vi "day 16 task 1.vi"   [LabVIEW 2019]
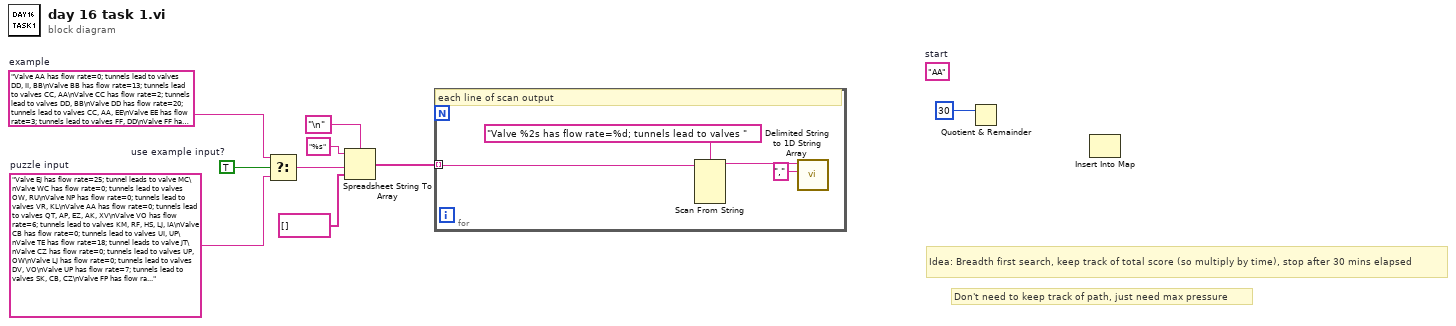
[diagram p0: block diagram]
diagram:
  (unwired) "AA"  # start
  w3 = TRUE  # use example input?
  w4 = "Valve EJ has flow rate=25; tunnel leads to valve MC\nValve WC has flow rate=0; tunnels lead to valves OW, RU\nValve NP has flow rate=0; tunnels lead to valves VR, KL\nValve AA has flow rate=0; tunnels lead to valves QT, AP, EZ, AK, XV\nValve VO has flow rate=6; tunnels lead to valves KM, RF, HS, LJ, IA\nValve CB has flow rate=0; tunnels lead to valves UI, UP\nValve TE has flow rate=18; tunnel leads to valve JT\nValve CZ has flow rate=0; tunnels lead to valves UP, OW\nValve LJ has flow rate=0; tunnels lead to valves DV, VO\nValve UP has flow rate=7; tunnels lead to valves SK, CB, CZ\nValve FP has flow rate=0; tunnels lead to valves OW, RE\nValve KM has flow rate=0; tunnels lead to valves SE, VO\nValve DV has flow rate=0; tunnels lead to valves LJ, UM\nValve FL has flow rate=0; tunnels lead to valves AH, TS\nValve VR has flow rate=24; tunnels lead to valves DM, TF, NP\nValve IA has flow rate=0; tunnels lead to valves VS, VO\nValve RF has flow rate=0; tunnels lead to valves VO, JF\nValve RT has flow rate=0; tunnels lead to valves UM, SE\nValve RU has flow rate=0; tunnels lead to valves AR, WC\nValve SE has flow rate=4; tunnels lead to valves GU, KM, CX, RT\nValve MC has flow rate=0; tunnels lead to valves EJ, AR\nValve TF has flow rate=0; tunnels lead to valves AH, VR\nValve CX has flow rate=0; tunnels lead to valves SE, TO\nValve GL has flow rate=11; tunnels lead to valves UY, KL, CY\nValve GU has flow rate=0; tunnels lead to valves SE, EZ\nValve VS has flow rate=0; tunnels lead to valves XN, IA\nValve EZ has flow rate=0; tunnels lead to valves AA, GU\nValve GK has flow rate=0; tunnels lead to valves FI, HZ\nValve JT has flow rate=0; tunnels lead to valves TE, XN\nValve DM has flow rate=0; tunnels lead to valves VR, HZ\nValve AR has flow rate=16; tunnels lead to valves UI, RU, MC\nValve XN has flow rate=9; tunnels lead to valves XP, JT, VS, GT, CY\nValve CY has flow rate=0; tunnels lead to valves XN, GL\nValve QT has flow rate=0; tunnels lead to valves UM, AA\nValve KL has flow rate=0; tunnels lead to valves GL, NP\nValve SK has flow rate=0; tunnels lead to valves XV, UP\nValve OW has flow rate=12; tunnels lead to valves CZ, WC, FP\nValve AK has flow rate=0; tunnels lead to valves AA, HS\nValve XV has flow rate=0; tunnels lead to valves AA, SK\nValve GT has flow rate=0; tunnels lead to valves XN, UM\nValve FI has flow rate=0; tunnels lead to valves JF, GK\nValve UY has flow rate=0; tunnels lead to valves JF, GL\nValve UM has flow rate=5; tunnels lead to valves DV, GT, RT, QT\nValve IQ has flow rate=0; tunnels lead to valves HZ, AH\nValve JF has flow rate=10; tunnels lead to valves RF, FI, UY, RE, TS\nValve TS has flow rate=0; tunnels lead to valves JF, FL\nValve AH has flow rate=23; tunnels lead to valves IQ, FL, TF\nValve HS has flow rate=0; tunnels lead to valves AK, VO\nValve HZ has flow rate=20; tunnels lead to valves IQ, DM, GK\nValve TO has flow rate=15; tunnel leads to valve CX\nValve XP has flow rate=0; tunnels lead to valves AP, XN\nValve AP has flow rate=0; tunnels lead to valves XP, AA\nValve RE has flow rate=0; tunnels lead to valves JF, FP\nValve UI has flow rate=0; tunnels lead to valves AR, CB"  # puzzle input
  w5 = "Valve AA has flow rate=0; tunnels lead to valves DD, II, BB\nValve BB has flow rate=13; tunnels lead to valves CC, AA\nValve CC has flow rate=2; tunnels lead to valves DD, BB\nValve DD has flow rate=20; tunnels lead to valves CC, AA, EE\nValve EE has flow rate=3; tunnels lead to valves FF, DD\nValve FF has flow rate=0; tunnels lead to valves EE, GG\nValve GG has flow rate=0; tunnels lead to valves FF, HH\nValve HH has flow rate=22; tunnel leads to valve GG\nValve II has flow rate=0; tunnels lead to valves AA, JJ\nValve JJ has flow rate=21; tunnel leads to valve II"  # example
  # "Don't need to keep track of path, just need max pressure"
  # "Idea: Breadth first search, keep track of total score (so multiply by time), stop after 30 mins elapsed"
  n1 = Select(t=w5, s=w3, f=w4) -> (s? t:f=w2:string)
  n2 = Spreadsheet String To Array(delimiter (Tab)="\n", format string="%s", spreadsheet string=w2, array type (2D Dbl)=string[] []) -> (array=w6:string[])
  n3 = for {
    tunnel: w6 -> [w13] mode=indexing
    # "each line of scan output"
    n4 = Scan From String(format string="Valve %2s has flow rate=%d; tunnels lead to valves ", input string=w13) -> (remaining string=w11:string)  [unwired: 6 in, 2 out]
    n5 = call <vilib>:"Delimited String to 1D String Array.vi"("delimiter"=",", "delimited string"=w11) -> ()  [unwired: 9 in, 1 out]
  }
  n6 = Quotient & Remainder(x=30 ("output 2")) -> ()  [unwired: 1 in, 2 out]
  n7 = Insert Into Map() -> ()  [unwired: 3 in, 3 out]
